vi "DSF.Engine.Framework.Create.Transfer Groups.vi"(8 "error in (no error)":errorcluster, 10 "Transfer Group Configurations":refnum<class "DSF.Shared.Configuration.Transfer Group.lvclass">[](array[class]), 11 "Framework in":refnum<class "DSF.Engine.Framework.lvclass">) -> (0 "error out":errorcluster, 2 "Transfer Groups":refnum<class "DSF.Engine.Transfer Group.lvclass">[](array[class]), 3 "Framework out":refnum<class "DSF.Engine.Framework.lvclass">)   [LabVIEW 2017, in "DSF.Engine.lvlib" / "DSF.Engine.Framework.lvclass"]
uses:
  DSF.Engine.Framework.lvclass
  Transfer/DSF.Engine.Transfer Group.lvclass
  Shared/Classes/Transfer Group/DSF.Shared.Configuration.Transfer Group.lvclass
  DSF.Engine.Framework.lvclass/DSF.Engine.Framework.ctl
  Cache/DSF.Engine.Memory.Cache.lvclass/DSF.Engine.Memory.Cache.ctl
  Shared/Classes/Transfer Group/DSF.Shared.Configuration.Transfer Group.lvclass/DSF.Shared.Configuration.Transfer Group.ctl
  Shared/Classes/Transfer/DSF.Shared.Configuration.Transfer.lvclass/DSF.Shared.Configuration.Transfer.ctl
  Pointer/DSF.Engine.Pointer.DBL.lvclass
  Timing/DSF.Engine.Timing.lvclass
  Cache/DSF.Engine.Memory.Cache.lvclass
  Shared/Classes/Transfer/DSF.Shared.Configuration.Transfer.lvclass
  Buffer/DSF.Engine.Memory.Buffer.lvclass
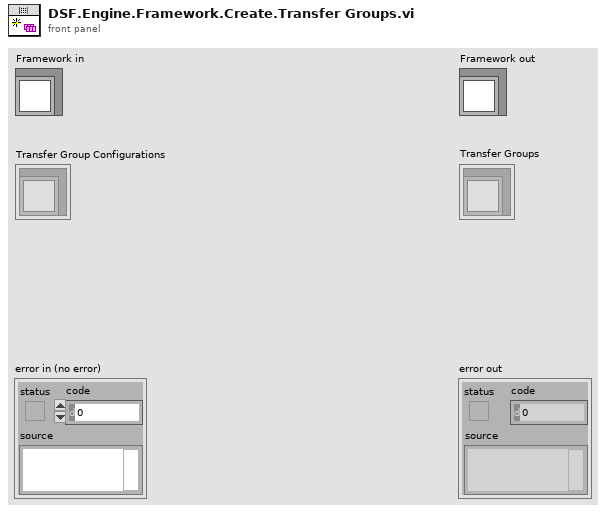
[diagram p1: front panel]
types:
  T1 = typedef "DSF Configuration API.lvlib/DSF Direction.ctl" = enum8{"Tx", "Rx"}
  T2 = typedef "DSF Configuration API.lvlib/DSF Timing Info.ctl" = cluster{"priority":u64, "decimation":u64, "offset":u64}
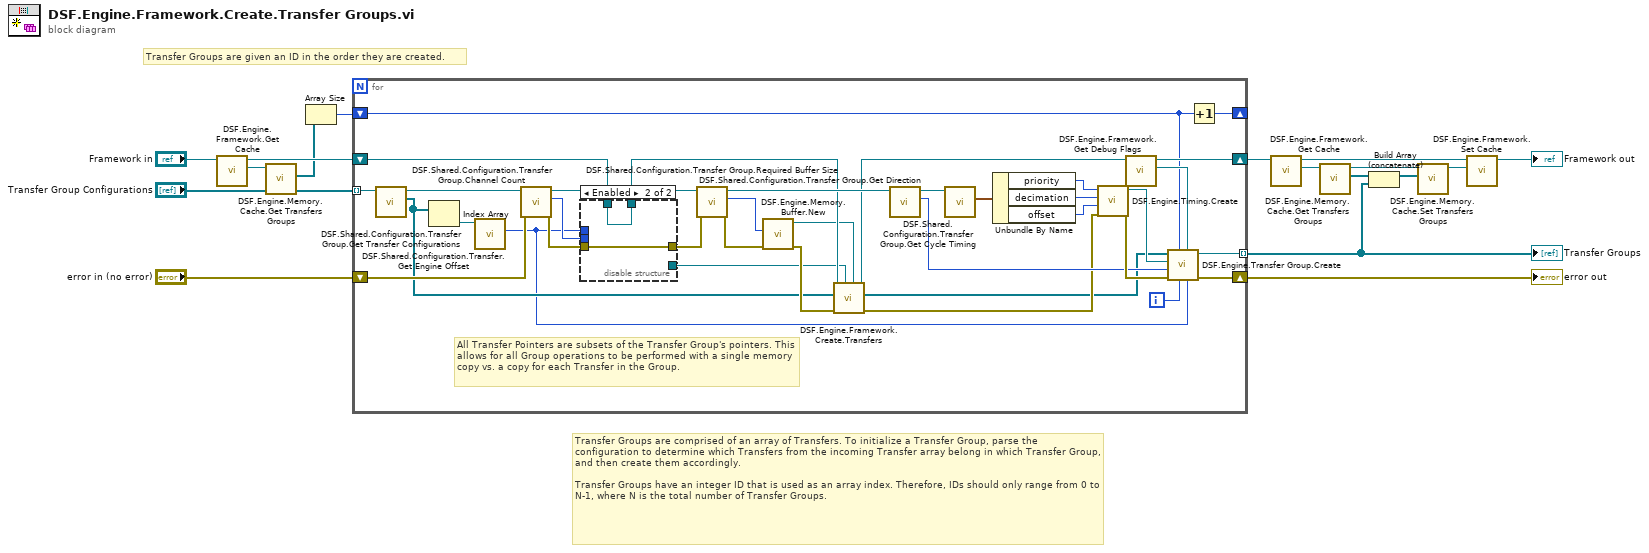
[diagram p0: block diagram]
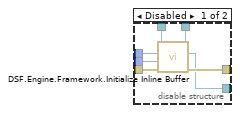
[diagram p2: hidden frame]
diagram:
  # "Transfer Groups are given an ID in the order they are created."
  # "Transfer Groups are comprised of an array of Transfers. To initialize a Transfer Group, parse the configuration to determine which Transfers from the incoming Transfer array belong in which Transfer Group, and then create them accordingly.\n\nTransfer Groups have an integer ID that is used as an array index. Therefore, IDs should only range from 0 to N-1, where N is the total number of Transfer Groups."
  n1 = call "DSF.Engine.Framework.Get Cache.vi"("Framework in"="Framework in") -> ("Cache"=w6:refnum<class "DSF.Engine.Memory.Cache.lvclass">, "Framework out"=w4:refnum<class "DSF.Engine.Framework.lvclass">)  [unwired: 9 in]
  n2 = call "DSF.Engine.Memory.Cache.Get Transfers Groups.vi"("Cache in"=w6) -> ("Transfers Groups"=w3:refnum<class "DSF.Engine.Transfer Group.lvclass">[])  [unwired: 9 in, 1 out]
  n3 = Array Size(array=w3) -> (size(s)=w16:i32)
  n4 = for {
    shift-right: [w52] -> w1
    shift-left: "error in (no error)" -> [w37]
    tunnel: [w38] -> w2 mode=indexing
    shift-right: [w42] -> w8
    shift-left: w4 -> [w35]
    shift-right: [w51] -> _
    shift-left: w16 -> [w40]
    tunnel: "Transfer Group Configurations" -> [w34] mode=indexing
    i -> [w39]
    # "All Transfer Pointers are subsets of the Transfer Group's pointers. This allows for all Group operations to be performed with a single memory copy vs. a copy for each Transfer in the Group."
    n5 = call "DSF.Shared.Configuration.Transfer Group.Get Transfer Configurations.vi"("Transfer Group Configuration in"=w34) -> ("Transfer Configurations"=w21:refnum<class "DSF.Shared.Configuration.Transfer.lvclass">[], "Transfer Group Configuration out"=w33:refnum<class "DSF.Shared.Configuration.Transfer Group.lvclass">)  [unwired: 9 in]
    n6 = Index Array(array=w21) -> (element=w32:refnum<class "DSF.Shared.Configuration.Transfer.lvclass">)  [unwired: 1 in]
    n7 = call "DSF.Shared.Configuration.Transfer.Get Engine Offset.vi"("Transfer Configuration in"=w32) -> ("engine offset"=w18:u64)  [unwired: 9 in, 1 out]
    n8 = call "DSF.Shared.Configuration.Transfer Group.Channel Count.vi"("error in (no error)"=w37, "Transfer Group Configuration in"=w33) -> ("error out"=w31:errorcluster, "total channel count"=w30:u64, "Transfer Group Configuration out"=w36:refnum<class "DSF.Shared.Configuration.Transfer Group.lvclass">)  [unwired: 7 in]
    n9 = disable-structure shown="Enabled" {
      disable-tunnel: w35 -> [w60 w61]
      disable-tunnel: w31 -> [w59 w62]
      disable-tunnel: w30 -> [w58 _]
      disable-tunnel: [w57 w62] -> w27
      disable-tunnel: [w56 w61] -> w23
      disable-tunnel: [w55 _] -> w19
      disable-tunnel: w18 -> [w54 _]
      frame Disabled {
        n10 = call-dynamic "DSF.Engine.Framework.Initialize Inline Buffer.vi"("error in (no error)"=w59, "channel count"=w58, "first channel offset"=w54, "Framework in"=w60) -> ("error out"=w57:errorcluster, "Buffer"=w55:refnum<class "DSF.Engine.Pointer.DBL.lvclass">, "Framework out"=w56:refnum<class "DSF.Engine.Framework.lvclass">)  [unwired: 5 in]
      }
      frame Enabled {
      }
    }
    n11 = call "DSF.Shared.Configuration.Transfer Group.Required Buffer Size.vi"("error in (no error)"=w27, "Transfer Group Configuration in"=w36) -> ("error out"=w28:errorcluster, "required buffer size"=w29:u64, "Transfer Group Configuration out"=w53:refnum<class "DSF.Shared.Configuration.Transfer Group.lvclass">)  [unwired: 7 in]
    n12 = call "DSF.Engine.Memory.Buffer.New.vi"("error in (no error)"=w28, "size"=w29) -> ("error out"=w26:errorcluster, "Buffer out"=w20:refnum<class "DSF.Engine.Memory.Buffer.lvclass">)  [unwired: 8 in]
    n13 = call "DSF.Engine.Framework.Create.Transfers.vi"("Group String Buffer"=w20, "Group Engine Buffer"=w19, "error in (no error)"=w26, "Transfer Configurations"=w21, "Framework in"=w23) -> ("error out"=w25:errorcluster, "Transfers"=w24:refnum<class "DSF.Engine.Transfer.lvclass">[], "Framework out"=w22:refnum<class "DSF.Engine.Framework.lvclass">)  [unwired: 4 in]
    n14 = call "DSF.Shared.Configuration.Transfer Group.Get Direction.vi"("Transfer Group Configuration in"=w53) -> ("direction"=w43:T1, "Transfer Group Configuration out"=w50:refnum<class "DSF.Shared.Configuration.Transfer Group.lvclass">)  [unwired: 9 in]
    n15 = call "DSF.Shared.Configuration.Transfer Group.Get Cycle Timing.vi"("Transfer Group Configuration in"=w50) -> ("cycle timing"=w49:T2)  [unwired: 9 in, 1 out]
    n16 = Unbundle By Name(w49) -> ("priority"=w45:u64, "decimation"=w46:u64, "offset"=w47:u64)
    n17 = call "DSF.Engine.Timing.Create.vi"("error in (no error)"=w25, "Offset"=w47, "Decimation"=w46, "Priority"=w45) -> ("error out"=w48:errorcluster, "Timing"=w44:refnum<class "DSF.Engine.Timing.lvclass">)  [unwired: 6 in]
    n18 = call "DSF.Engine.Framework.Get Debug Flags.vi"("Framework in"=w22) -> ("Debug Flags"=w41:refnum<class "DSF.Engine.Debug Flags.lvclass">, "Framework out"=w42:refnum<class "DSF.Engine.Framework.lvclass">)  [unwired: 9 in]
    n19 = call "DSF.Engine.Transfer Group.Create.vi"("engine offset"=w18, "Debug Flags"=w41, "transceiver id"=w39, "framework id"=w40, "error in (no error)"=w48, "Direction"=w43, "Timing"=w44, "Transfers"=w24) -> ("error out"=w52:errorcluster, "Transfer Group out"=w38:refnum<class "DSF.Engine.Transfer Group.lvclass">)  [unwired: 2 in]
    n20 = Increment(x=w40) -> (x+1=w51:i32)
  }
  "error out" <- w1
  "Transfer Groups" <- w2
  n21 = call "DSF.Engine.Framework.Get Cache.vi"("Framework in"=w8) -> ("Cache"=w13:refnum<class "DSF.Engine.Memory.Cache.lvclass">, "Framework out"=w14:refnum<class "DSF.Engine.Framework.lvclass">)  [unwired: 9 in]
  n22 = call "DSF.Engine.Memory.Cache.Get Transfers Groups.vi"("Cache in"=w13) -> ("Transfers Groups"=w10:refnum<class "DSF.Engine.Transfer Group.lvclass">[], "Cache out"=w11:refnum<class "DSF.Engine.Memory.Cache.lvclass">)  [unwired: 9 in]
  n23 = Build Array (concatenate)(w10, w2) -> (w9:refnum<class "DSF.Engine.Transfer Group.lvclass">[])
  n24 = call "DSF.Engine.Memory.Cache.Set Transfers Groups.vi"("Transfers Groups"=w9, "Cache in"=w11) -> ("Cache out"=w12:refnum<class "DSF.Engine.Memory.Cache.lvclass">)  [unwired: 9 in]
  n25 = call "DSF.Engine.Framework.Set Cache.vi"("Cache"=w12, "Framework in"=w14) -> ("Framework out"=→"Framework out":refnum<class "DSF.Engine.Framework.lvclass">)  [unwired: 9 in]
